vi "Set Response to Error.vi"(8 "error in (no error)":errorcluster, 10 "response":T1, 11 "Error Handler in":refnum<class "Error Handler.lvclass">) -> (0 "error out":errorcluster, 3 "Error Handler out":refnum<class "Error Handler.lvclass">)   [LabVIEW 2021, in "Error Handler.lvlib" / "Error Handler.lvclass"]
uses:
  Error Handler.lvclass
  Error Handler.lvclass/Error Handler.ctl
  public types/response.ctl
  Error Handler.lvlib
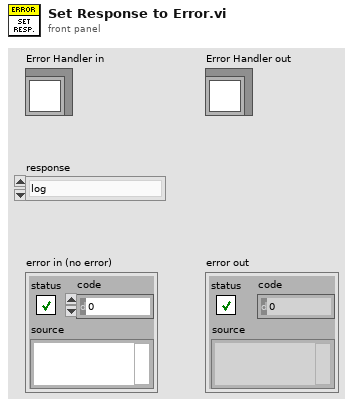
[diagram p1: front panel]
types:
  T1 = typedef "Error Handler.lvlib/response.ctl" = enum16{"log", "log & popup", "log & exit", "log & popup & exit", "popup", "popup & exit", "exit", "ignore"}
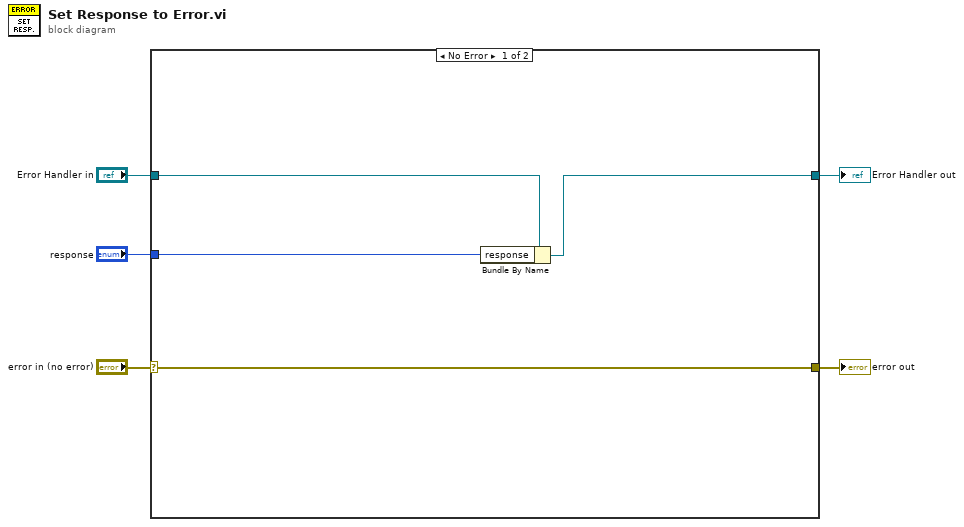
[diagram p0: block diagram]
diagram:
  n1 = case shown="No Error" "error in (no error)" {
    selector: "error in (no error)" -> [w8 w11]
    tunnel: [w8 w11] -> w4
    tunnel: [w7 w10] -> w2
    tunnel: "Error Handler in" -> [w9 w10]
    tunnel: "response" -> [w6 _]
    frame No Error {
      n2 = Bundle By Name(cluster=w9, "response"=w6) -> (w7:refnum<class "Error Handler.lvclass">)
    }
    frame Error {
    }
  }
  "error out" <- w4
  "Error Handler out" <- w2
